vi "IMAQ DLL Test.vi"() -> ()   [LabVIEW 2016]
uses:
  x64/Release/LabView IMAQ Images.dll
panel:
  out "LV Not Zero No.":i32
  out "Just Not Zero":u16
  out "Linear Indicies":i32[](array[numeric])
  out "notZeroCols":i32[](array[numeric])
  out "numNotZero":u16
  out "X Resolution":i32
  out "Y Resolution":i32
  in  "Input Data":u16[][](array[numeric])
  out "notZeroRows":i32[](array[numeric])
  out "Image Pixels (U16)":u16[][](array[numeric])
  out "Pixel Size (Bytes)":i32
  out "LineWidth(Pixels)":i32
  out "Pixel Pointer out":u64 format="%.6f"
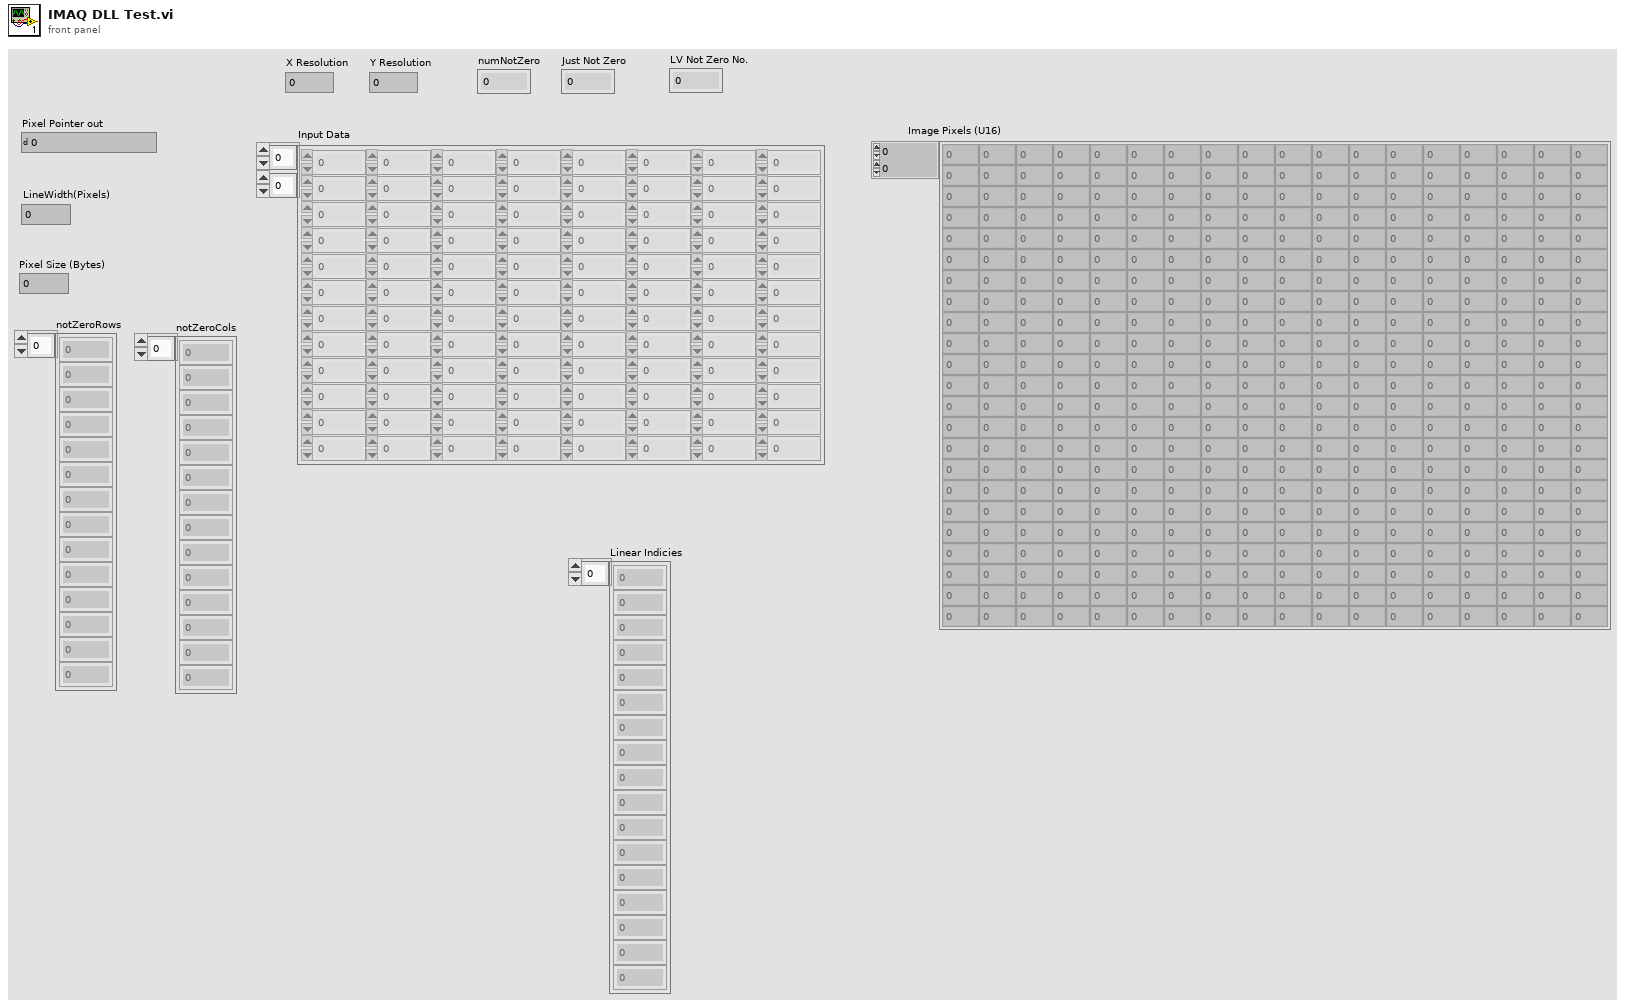
[diagram p1: front panel]
types:
  T1 = enum32{"Map Pixel Pointer", "Unmap Pixel Pointer", "Get Pixels Infos"}
  T2 = typedef "Image Type" = u32
  T3 = typedef "IMAQ Image.ctl" = refnum<image>
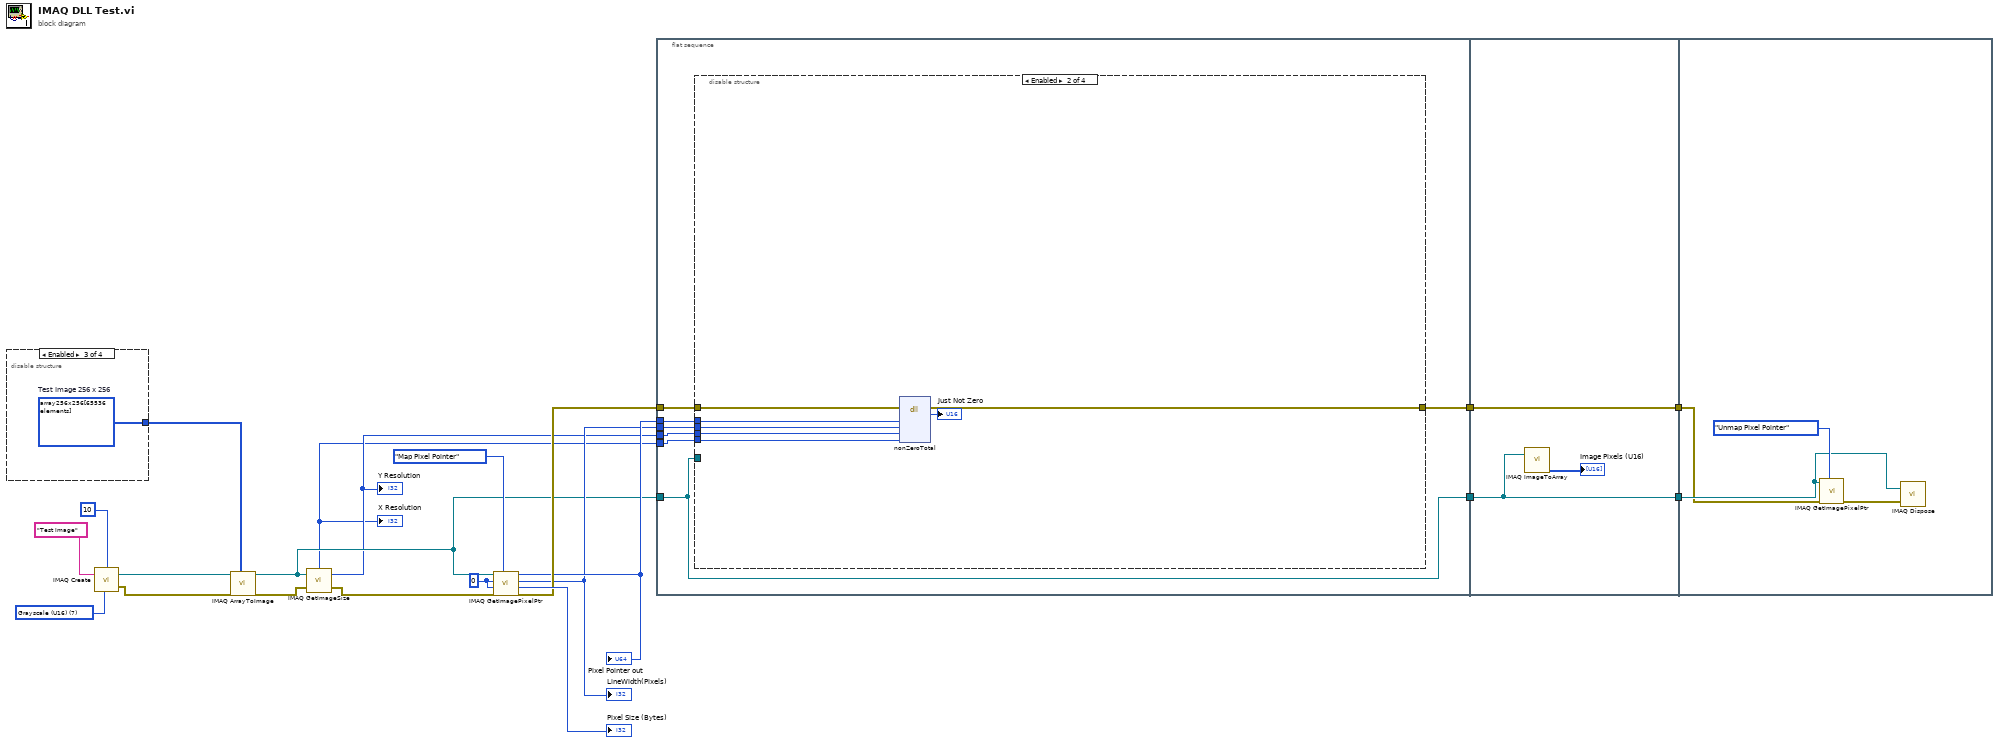
[diagram p0: block diagram]
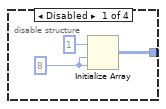
[diagram p2: hidden frame]
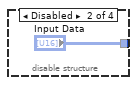
[diagram p3: hidden frame]
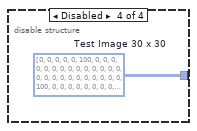
[diagram p4: hidden frame]
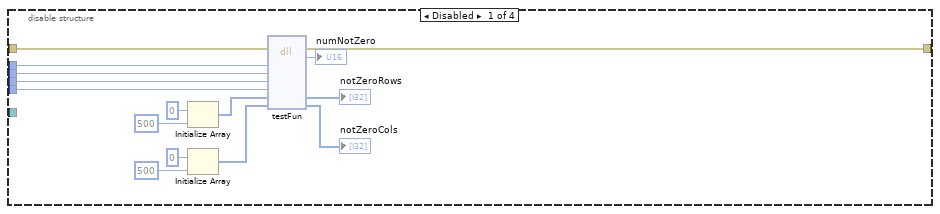
[diagram p5: hidden frame]
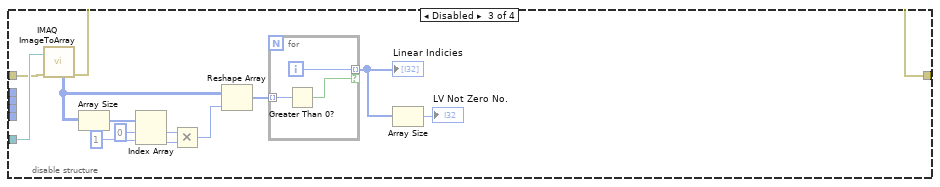
[diagram p6: hidden frame]
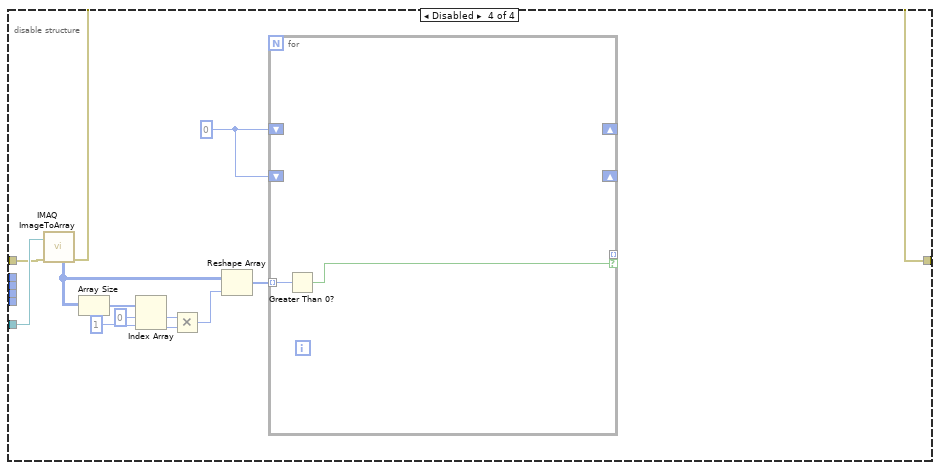
[diagram p7: hidden frame]
diagram:
  w17 = 0 ("X Coordinate")
  w20 = T2 7 items=["Grayscale (U8)", "Grayscale (I16)", "Grayscale (SGL)", "Complex (CSG)", "RGB (U32)", "HSL (U32)", "RGB (U64)", "Grayscale (U16)"] ("Image Type")
  n1 = disable-structure shown="Enabled" {
    disable-tunnel: [w23 "Input Data" w26 w27] -> w1
    frame Disabled {
      w22 = 8 ("dimension size")
      n2 = Initialize Array(u16 1 ("element"), w22, w22) -> (w23:u16[][])
    }
    frame Disabled {
    }
    frame Enabled {
      w26 = u16[][] array256x256[65536 elements]  # Test Image 256 x 256
    }
    frame Disabled {
      w27 = u16[][] [[0, 0, 0, 0, 0, 100, 0, 0, 0, 0, 0, 0, 0, 0, 0, 0, 0, 0, 0, 0, 0, 0, 0, 0, 0, 0, 0, 0, 0, 0], [0, 100, 0, 0, 0, 0, 0, 0, 0, 0, 0, 0, 0, 0, 0, 0, 0, 0, 0, 0, 0, 0, 0, 0, 0, 0, 0, 0, 0, 0], [0, 0, 0, 0, 0, 100, 0, 0, 0, 0, 0, 0, 0, 0, 0, 0, 0, 100, 0, 0, 0, 0, 0, 0, 0, 0, 0, 0, 0, 0], [0, 0, 0, 0, 0, 100, 0, 0, 0, 0, 0, 0, 0, 0, 0, 0, 0, 0, 0, 0, 0, 0, 0, 0, 0, 0, 0, 0, 0, 0], [0, 0, 0, 0, 0, 0, 0, 0, 0, 0, 0, 0, 0, 0, 0, 0, 0, 0, 0, 0, 0, 0, 0, 0, 0, 0, 0, 0, 0, 0], [0, 0, 0, 0, 0, 0, 0, 0, 0, 0, 0, 0, 0, 0, 0, 0, 0, 0, 0, 0, 0, 0, 0, 0, 0, 0, 0, 0, 0, 0], [0, 0, 0, 0, 0, 0, 0, 0, 100, 0, 0, 100, 0, 0, 0, 0, 0, 0, 0, 100, 0, 0, 0, 0, 0, 0, 0, 0, 100, 0], [0, 0, 0, 0, 100, 100, 0, 0, 0, 0, 0, 0, 0, 0, 0, 0, 0, 0, 0, 0, 0, 0, 0, 0, 0, 0, 0, 0, 0, 0], [0, 0, 0, 0, 0, 0, 0, 0, 0, 0, 0, 0, 0, 0, 0, 100, 0, 0, 0, 0, 0, 0, 0, 0, 0, 0, 0, 0, 0, 0], [0, 0, 0, 0, 0, 100, 0, 0, 0, 0, 0, 0, 0, 0, 0, 0, 0, 0, 0, 0, 0, 0, 100, 0, 0, 0, 0, 0, 0, 100], [0, 0, 0, 0, 0, 0, 0, 0, 0, 0, 0, 0, 0, 0, 0, 0, 0, 0, 0, 0, 0, 100, 0, 0, 0, 0, 0, 0, 0, 0], [0, 100, 0, 0, 0, 0, 0, 0, 0, 0, 0, 0, 0, 0, 0, 0, 100, 0, 0, 0, 0, 0, 100, 0, 0, 0, 0, 0, 0, 0], [0, 0, 0, 0, 0, 0, 0, 0, 0, 0, 0, 0, 0, 0, 0, 0, 0, 0, 0, 0, 0, 0, 0, 0, 0, 0, 0, 0, 0, 0], [0, 0, 0, 0, 0, 0, 0, 0, 0, 0, 0, 0, 0, 0, 0, 0, 0, 0, 0, 100, 0, 0, 0, 0, 0, 0, 0, 0, 0, 0], [0, 0, 0, 0, 0, 0, 0, 0, 0, 0, 0, 0, 0, 0, 0, 0, 0, 0, 0, 0, 0, 0, 0, 0, 100, 0, 0, 0, 0, 0], [0, 0, 0, 0, 0, 0, 100, 0, 0, 0, 0, 0, 0, 0, 0, 0, 0, 0, 0, 0, 0, 0, 0, 0, 0, 0, 0, 0, 100, 0], [0, 0, 0, 0, 0, 0, 0, 0, 0, 0, 0, 0, 0, 0, 100, 0, 0, 0, 0, 0, 0, 0, 0, 0, 0, 0, 0, 0, 0, 0], [0, 0, 0, 0, 0, 0, 0, 0, 0, 0, 0, 0, 0, 0, 0, 0, 0, 0, 0, 0, 0, 0, 0, 0, 0, 0, 0, 0, 0, 0], [0, 0, 0, 0, 0, 0, 0, 0, 0, 0, 0, 0, 0, 0, 0, 0, 0, 0, 100, 0, 0, 0, 0, 0, 0, 0, 0, 0, 0, 0], [0, 0, 0, 0, 0, 0, 0, 0, 0, 0, 0, 0, 0, 0, 0, 0, 0, 0, 0, 0, 0, 0, 0, 0, 0, 100, 0, 0, 0, 0], [0, 0, 0, 0, 0, 0, 0, 0, 0, 0, 100, 0, 0, 0, 0, 0, 0, 0, 0, 0, 0, 0, 0, 0, 0, 0, 0, 100, 100, 0], [100, 0, 0, 0, 0, 0, 0, 0, 0, 0, 0, 0, 0, 0, 0, 0, 0, 0, 0, 0, 0, 0, 0, 0, 0, 0, 0, 0, 0, 100], [100, 0, 0, 0, 0, 0, 0, 0, 0, 0, 0, 0, 0, 0, 0, 0, 0, 0, 0, 0, 0, 100, 0, 0, 0, 0, 0, 0, 0, 0], [0, 0, 0, 0, 0, 0, 0, 0, 0, 0, 0, 100, 100, 0, 0, 0, 0, 0, 0, 0, 0, 0, 0, 0, 0, 0, 0, 0, 0, 0], [0, 0, 0, 0, 0, 0, 0, 0, 0, 0, 0, 0, 0, 0, 0, 0, 0, 0, 0, 0, 0, 0, 0, 0, 0, 0, 0, 0, 100, 0], [0, 0, 0, 0, 0, 0, 0, 0, 0, 0, 0, 0, 0, 0, 0, 0, 0, 0, 0, 0, 0, 0, 0, 0, 0, 0, 0, 0, 0, 0], [0, 0, 0, 0, 0, 0, 0, 100, 0, 0, 0, 0, 0, 0, 0, 100, 0, 0, 0, 0, 0, 0, 0, 0, 0, 0, 0, 0, 0, 0], [0, 0, 0, 0, 0, 0, 0, 0, 0, 0, 0, 0, 0, 0, 0, 0, 0, 0, 0, 0, 0, 0, 0, 0, 0, 0, 0, 0, 0, 0], [0, 0, 0, 0, 0, 0, 0, 0, 0, 0, 0, 0, 0, 0, 0, 0, 0, 0, 0, 0, 0, 0, 0, 0, 0, 0, 0, 0, 0, 0], [0, 0, 0, 0, 0, 0, 0, 0, 0, 0, 0, 0, 0, 0, 0, 0, 0, 0, 0, 0, 0, 0, 0, 0, 0, 0, 0, 0, 0, 0]]  # Test Image 30 x 30
    }
  }
  n3 = call "IMAQ Create"("Border Size"=10, "Image Name"="Test Image", "Image Type"=w20) -> ("New Image"=w15:T3, "error out"=w14:errorcluster)  [unwired: 2 in]
  n4 = call "IMAQ ArrayToImage"("Image Pixels (U16)"=w1, "error in (no error)"=w14, "Image"=w15) -> ("error out"=w6:errorcluster, "Image Out"=w4:T3)  [unwired: 7 in]
  n5 = call "IMAQ GetImageSize"("Image"=w4, "error in (no error)"=w6) -> ("Y Resolution"=w3:i32, "X Resolution"=w2:i32, "error out"=w5:errorcluster)  [unwired: 2 in]
  "Y Resolution" <- w3
  "X Resolution" <- w2
  n6 = call "IMAQ GetImagePixelPtr"("Function"=T1."Map Pixel Pointer", "error in (no error)"=w5, "Y Coordinate"=w17, "X Coordinate"=w17, "Image"=w4) -> ("error out"=w13:errorcluster, "Pixel Size (Bytes)"=→"Pixel Size (Bytes)":i32, "LineWidth(Pixels)"=w7:i32, "Pixel Pointer out"=w12:u64)  [unwired: 1 in, 2 out]
  "Pixel Pointer out" <- w12
  "LineWidth(Pixels)" <- w7
  n7 = flat-sequence {
    tunnel: w13 -> [w34]
    tunnel: w12 -> [w33]
    tunnel: [w32] -> w11
    tunnel: w4 -> [w28]
    tunnel: [w28] -> w9
    tunnel: w7 -> [w31]
    tunnel: w3 -> [w30]
    tunnel: w2 -> [w29]
    tunnel: w11 -> [w89]
    tunnel: [w89] -> w10
    tunnel: w9 -> [w88]
    tunnel: [w88] -> w8
    tunnel: w10 -> [w90]
    tunnel: w8 -> [w91]
    frame #0 {
      n8 = disable-structure shown="Enabled" {
        disable-tunnel: w34 -> [w49 w56 w68 w83]
        disable-tunnel: w33 -> [w48 w55 _ _]
        disable-tunnel: [w47 w54 w60 w75] -> w32
        disable-tunnel: w31 -> [w46 w53 _ _]
        disable-tunnel: w30 -> [w45 w52 _ _]
        disable-tunnel: w29 -> [w44 w51 _ _]
        disable-tunnel: w28 -> [_ _ w69 w84]
        frame Disabled {
          n9 = Initialize Array(0 ("element"), 500 ("dimension size")) -> (w41:i32[])
          n10 = Initialize Array(0 ("element"), 500 ("dimension size")) -> (w36:i32[])
          n11 = dll-call lib="D:/Microscope-Control/Tools/LabView IMAQ Images/LabView IMAQ Images DLL Files/x64/Release/LabView IMAQ Images.dll" fn="testFun"(error in=w49, "imPointer"=w48, "LV_Line_Width"=w46, "LV_Rows"=w45, "LV_Cols"=w44, "notZeroRows"=w41, "notZeroCols"=w36) -> (error out=w47:errorcluster, "numNotZero"=→"numNotZero":u16, "notZeroRows"=→"notZeroRows":i32[], "notZeroCols"=→"notZeroCols":i32[])  [unwired: 6 in, 1 out]
        }
        frame Enabled {
          n12 = dll-call lib="D:/Microscope-Control/Tools/LabView IMAQ Images/LabView IMAQ Images DLL Files/x64/Release/LabView IMAQ Images.dll" fn="nonZeroTotal"(error in=w56, "imPointer"=w55, "LV_Line_Width"=w53, "LV_Rows"=w52, "LV_Cols"=w51) -> (error out=w54:errorcluster, "numNotZero"=→"Just Not Zero":u16)  [unwired: 6 in, 1 out]
        }
        frame Disabled {
          n13 = call "IMAQ ImageToArray"("error in (no error)"=w68, "Image"=w69) -> ("Image Pixels (U16)"=w63:u16[][], "error out"=w60:errorcluster)  [unwired: 2 in, 3 out]
          n14 = Array Size(array=w63) -> (size(s)=w64:i32[])
          n15 = Index Array(array=w64, index #1=0 ("index"), index #2=1 ("index")) -> (element #1=w67:i32, element #2=w62:i32)
          n16 = Multiply(x=w67, y=w62) -> (x*y=w61:i32)
          n17 = Reshape Array(w63, w61) -> (w59:u16[])
          n18 = for {
            tunnel: w59 -> [w72] mode=indexing
            tunnel: [w71] -> w58 mode=indexing if=w70
            i -> [w71]
            n19 = Greater Than 0?(x=w72) -> (x > 0?=w70:bool)
          }
          "Linear Indicies" <- w58
          n20 = Array Size(array=w58) -> (size(s)=→"LV Not Zero No.":i32)
        }
        frame Disabled {
          w73 = 0
          n21 = call "IMAQ ImageToArray"("error in (no error)"=w83, "Image"=w84) -> ("Image Pixels (U16)"=w78:u16[][], "error out"=w75:errorcluster)  [unwired: 2 in, 3 out]
          n22 = Array Size(array=w78) -> (size(s)=w79:i32[])
          n23 = Index Array(array=w79, index #1=0 ("index"), index #2=1 ("index")) -> (element #1=w82:i32, element #2=w77:i32)
          n24 = Multiply(x=w82, y=w77) -> (x*y=w76:i32)
          n25 = Reshape Array(w78, w76) -> (w74:u16[])
          n26 = for {
            tunnel: w74 -> [w86] mode=indexing
            tunnel: _ -> [_] mode=indexing if=w85
            shift-right: _ -> [_]
            shift-left: w73 -> [_]
            shift-right: _ -> [_]
            shift-left: w73 -> [_]
            n27 = Greater Than 0?(x=w86) -> (x > 0?=w85:bool)
          }
        }
      }
    }
    frame #1 {
      n28 = call "IMAQ ImageToArray"("Image"=w88) -> ("Image Pixels (U16)"=→"Image Pixels (U16)":u16[][])  [unwired: 3 in, 4 out]
    }
    frame #2 {
      n29 = call "IMAQ GetImagePixelPtr"("Function"=T1."Unmap Pixel Pointer", "error in (no error)"=w90, "Image"=w91) -> ("error out"=w92:errorcluster)  [unwired: 3 in, 5 out]
      n30 = call "IMAQ Dispose"("Image"=w91, "error in (no error)"=w92) -> ()  [unwired: 4 in, 1 out]
    }
  }
